vi "Lightning Teleop.vi"() -> ()   [LabVIEW 2014]
uses:
  Global Objects.vi
panel:
  out "error out":errorcluster
  in  "error in":errorcluster
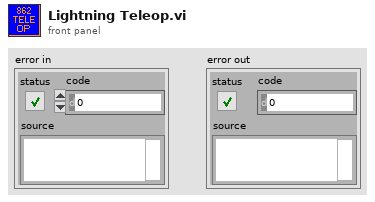
[diagram p1: front panel]
types:
  T1 = typedef "Teleop Commands.ctl" = cluster{"Throttle":dbl, "Turn":dbl, "Up Shift Commanded":bool, "Down Shift Commanded":bool}
  T2 = typedef "Joystick Info.ctl" = cluster{"JoystickDevRef":T3}
  T3 = typedef "WPI_JoystickDevRef.ctl" = cluster{"Device":T4}
  T4 = typedef "WPI_JoystickDeviceEnum.ctl" = enum16{"USB 0", "USB 1", "USB 2", "USB 3", "USB 4", "USB 5"}
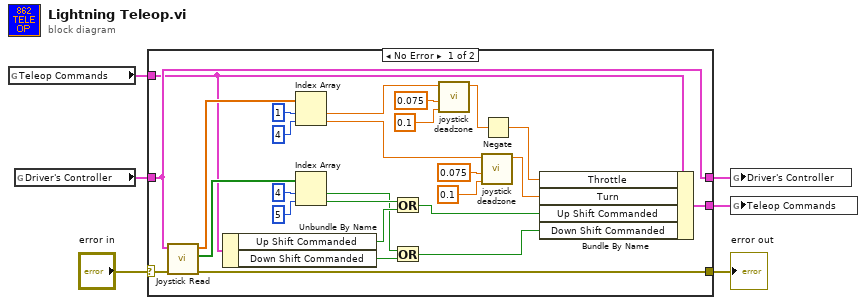
[diagram p0: block diagram]
diagram:
  n1 = global read "Global Objects.vi" "Teleop Commands"() -> (w2:T1)
  n2 = global read "Global Objects.vi" "Driver's Controller"() -> (w4:T2)
  n3 = case shown="No Error" "error in" {
    selector: "error in" -> [w31 w35]
    tunnel: [w30 w35] -> w5
    tunnel: [w32 w34] -> w3
    tunnel: w4 -> [w32 w34]
    tunnel: w2 -> [w14 w33]
    tunnel: [w23 w33] -> w1
    frame No Error {
      n4 = call "Joystick Read.vi"("error in"=w31, "Joystick In"=w32) -> ("error out"=w30:errorcluster, "Buttons"=w17:bool[], "Axes"=w29:dbl[])  [unwired: 6 in, 1 out]
      n5 = Unbundle By Name(w14) -> ("Up Shift Commanded"=w13:bool, "Down Shift Commanded"=w9:bool)
      n6 = Index Array(array=w29, index #1=1 ("index"), index #2=4 ("index")) -> (element #1=w27:dbl, element #2=w19:dbl)
      n7 = Index Array(array=w17, index #1=4 ("index"), index #2=5 ("index")) -> (element #1=w10:bool, element #2=w12:bool)
      n8 = Or(x=w12, y=w13) -> (x .or. y?=w11:bool)
      n9 = Or(x=w10, y=w9) -> (x .or. y?=w8:bool)
      n10 = call "joystick deadzone.vi"("minpower"=0.1, "deadzone"=0.075, "joystick"=w27) -> ("joyout"=w24:dbl)  [unwired: 8 in]
      n11 = call "joystick deadzone.vi"("minpower"=0.1, "deadzone"=0.075, "joystick"=w19) -> ("joyout"=w18:dbl)  [unwired: 8 in]
      n12 = Negate(x=w24) -> (-x=w7:dbl)
      n13 = Bundle By Name(cluster=w14, "Throttle"=w7, "Turn"=w18, "Up Shift Commanded"=w11, "Down Shift Commanded"=w8) -> (w23:T1)
    }
    frame Error {
    }
  }
  "error out" <- w5
  n14 = global write "Global Objects.vi" "Driver's Controller"(w3) -> ()
  n15 = global write "Global Objects.vi" "Teleop Commands"(w1) -> ()
